vi "excel data log.vi"() -> ()   [LabVIEW 2017]
uses:
  <instrlib>/Agilent 3446X Series/Public/Data/Read (Single Point).vi
  <instrlib>/Agilent 3446X Series/Agilent 3446X Series.lvlib
panel:
  out "Waveform Chart":dbl(graph)
  in  "VISA resource name":refnum<visa-resource-name>
  in  "Auto Range (T: Enable)":bool=TRUE
  in  "Measurement Function (10: Voltage DC)":i32(ring)=10 items=["Continuity", "Current AC", "Current DC", "Diode", "Frequency", "Resistance 4-wire", "Period", "Resistance 2-wire", "Temperature", "Voltage AC", "Voltage DC", "Voltage DC Ratio"]
  out "Measurement":dbl
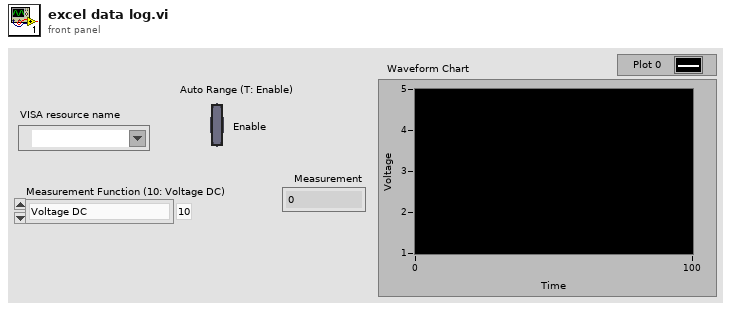
[diagram p1: front panel]
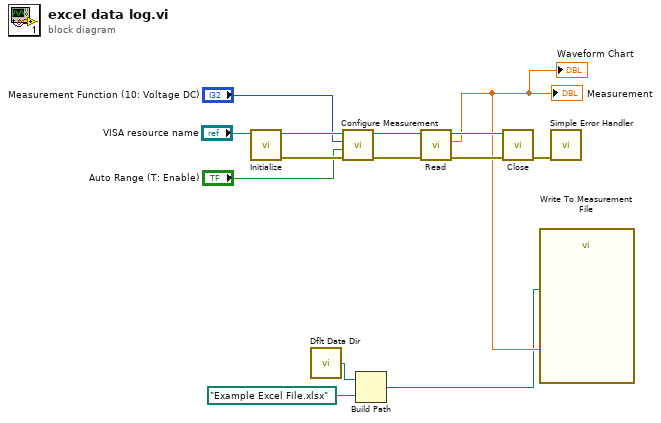
[diagram p0: block diagram]
diagram:
  n1 = call <instrlib>:"Initialize.vi"("VISA resource name"="VISA resource name") -> ("error out"=w12:errorcluster, "VISA resource name out"=w13:refnum<visa-resource-name>)  [unwired: 4 in, 5 out]
  n2 = call <vilib>:"Dflt Data Dir.vi"() -> ("App:Default Data Directory"=w3:path)
  n3 = call <instrlib>:"Configure Measurement.vi"("error in (no error)"=w12, "Auto Range (T: Enable)"="Auto Range (T: Enable)", "Measurement Function (10: Voltage DC)"="Measurement Function (10: Voltage DC)", "VISA resource name"=w13) -> ("error out"=w8:errorcluster, "VISA resource name out"=w9:refnum<visa-resource-name>)  [unwired: 2 in, 4 out]
  n4 = Build Path(base path=w3, name or relative path=path "Example Excel File.xlsx" ("default name")) -> (appended path=w1:path)
  n5 = call-poly <instrlib>:"Read.vi"("error in (no error)"=w8, "VISA resource name"=w9) -> ("error out"=w11:errorcluster, "Measurement"=w4:dbl, "VISA resource name out"=w10:refnum<visa-resource-name>)  [unwired: 7 out]
  "Measurement" <- w4
  "Waveform Chart" <- w4
  n6 = call <instrlib>:"Close.vi"("error in (no error)"=w11, "VISA resource name"=w10) -> ("error out"=w14:errorcluster)  [unwired: 9 out]
  n7 = call "Write To Measurement File"("Signals"=w4, "Filename"=w1) -> ()  [unwired: 15 in, 3 out]
  n8 = call <vilib>:"Simple Error Handler.vi"("error in (no error)"=w14) -> ()  [unwired: 1 in, 8 out]
